vi "2015HEWH_ParseERDInfo.vi"(8 "Error In":errorcluster, 9 "Disable Electronic Mixing Valve (EMV) List":bool, 10 "Disable ERD (Main)":bool, 11 "ERD Data Out":T4[](array[typedef]) {"ERD Number" format="%.0x"}) -> (0 "Error Out":errorcluster, 3 "ERD Data":T1 {"ERD Therm Data"."EEV Possition" format="%0.0f"; "ERD Therm Data"."T6" format="%.1f"; "ERD Therm Data"."T2" format="%.1f"; "ERD Therm Data"."T3a" format="%.1f"; "ERD Therm Data"."T3b" format="%.1f"; "ERD Therm Data"."T4" format="%.1f"; "ERD Therm Data"."T5" format="%.1f"; "ERD Therm Data"."Current" format="%.1f"})   [LabVIEW 2016]
uses:
  type defs/ERD Read Data Out.ctl
  type defs/HEWH ERD Data.ctl
  type defs/HEWH Faults.ctl
  type defs/HEWH Mixing Valve.ctl
  library/GEA2_Toolkit.lvlib
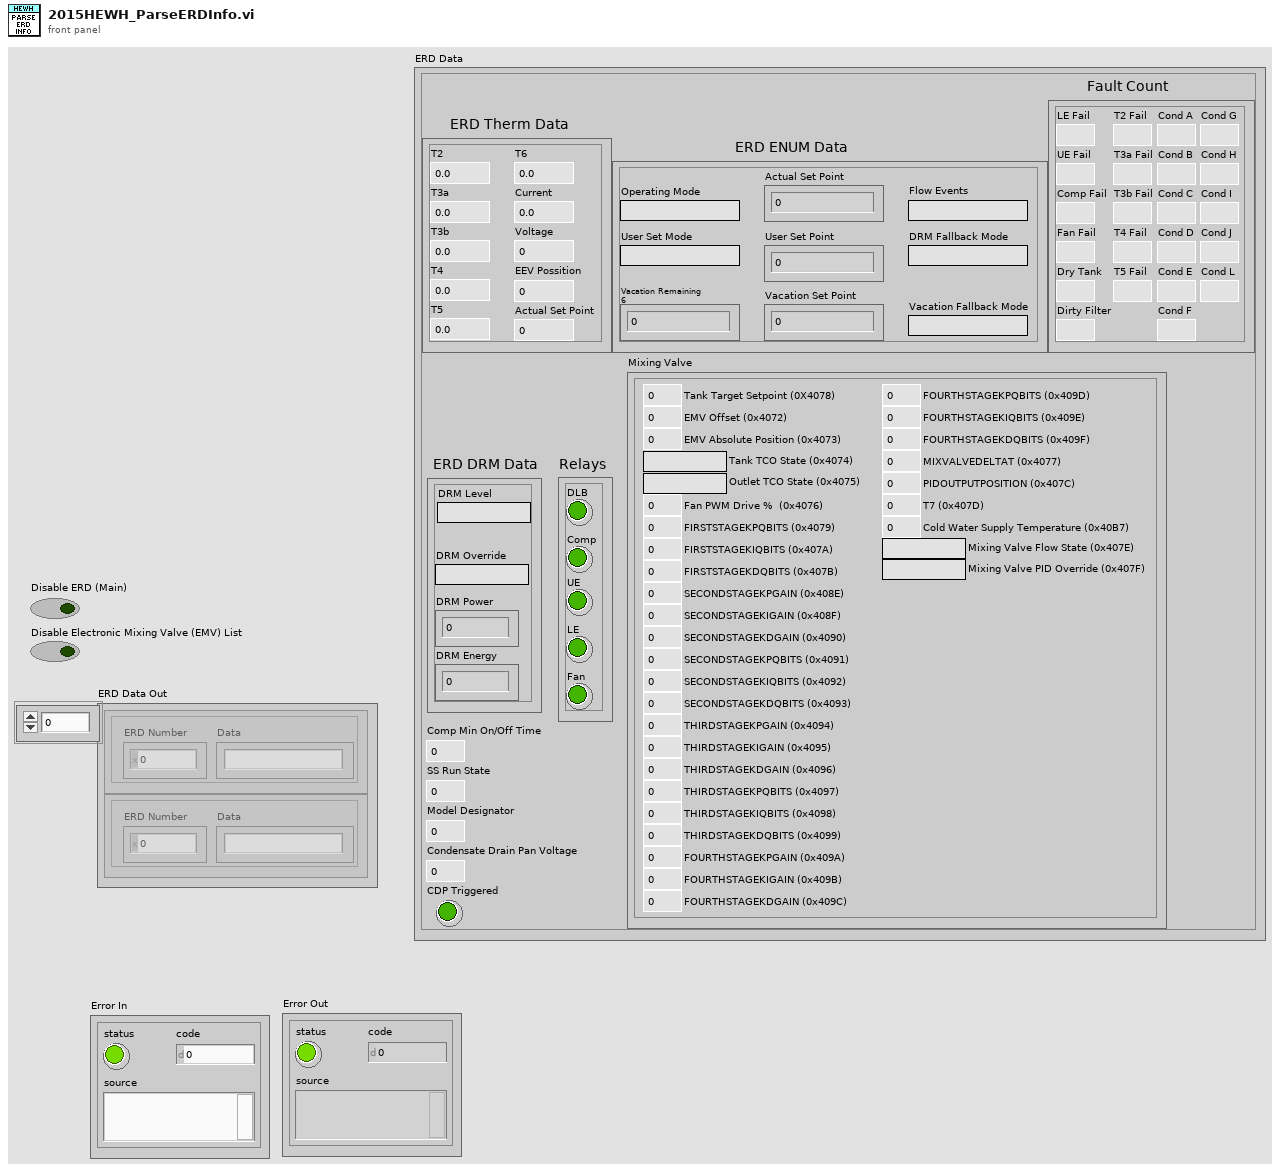
[diagram p1: front panel]
types:
  T1 = typedef "HEWH ERD Data.ctl" = cluster{"ERD Therm Data":cluster{"T2":dbl, "T3a":dbl, "T3b":dbl, "T4":dbl, "T5":dbl, "T6":dbl, "Current":dbl, "Voltage":dbl, "EEV Possition":dbl, "Actual Set Point":dbl}, "ERD ENUM Data":cluster{"Actual Set Point":dbl, "Flow Events":string, "User Set Mode":string, "Operating Mode":string, "DRM Fallback Mode":string, "Vacation Fallback Mode":string, "User Set Point":dbl, "Vacation Set Point":dbl, "Vacation Remaining\n6":dbl}, "ERD DRM Data":cluster{"DRM Level":string, "DRM Override":string, "DRM Power":dbl, "DRM Energy":dbl}, "Fault Count":T2, "Relays":cluster{"DLB":bool, "Comp":bool, "UE":bool, "LE":bool, "Fan":bool}, "Comp Min On/Off Time":u16, "SS Run State":u16, "Condensate Drain Pan Voltage":u16, "CDP Triggered":bool, "Model Designator":u8, "Mixing Valve":T3}
  T2 = typedef "HEWH Faults.ctl" = cluster{"LE Fail":u32, "UE Fail":u32, "Comp Fail":u32, "T2 Fail":u32, "T3a Fail":u32, "T3b Fail":u32, "T4 Fail":u32, "T5 Fail":u32, "Cond A":u32, "Cond B":u32, "Cond C":u32, "Cond D":u32, "Cond E":u32, "Cond F":u32, "Cond G":u32, "Cond H":u32, "Cond I":u32, "Cond J":u32, "Cond L":u32, "Fan Fail":u32, "Dirty Filter":u32, "Dry Tank":u32}
  T3 = typedef "HEWH Mixing Valve.ctl" = cluster{"Tank Target Setpoint (0X4078)":dbl, "EMV Offset (0x4072)":dbl, "EMV Absolute Position (0x4073)":dbl, "Tank TCO State (0x4074)":string, "Outlet TCO State (0x4075)":string, "Fan PWM Drive %  (0x4076)":dbl, "FIRSTSTAGEKPQBITS (0x4079)":dbl, "FIRSTSTAGEKIQBITS (0x407A)":dbl, "FIRSTSTAGEKDQBITS (0x407B)":dbl, "SECONDSTAGEKPGAIN (0x408E)":dbl, "SECONDSTAGEKIGAIN (0x408F)":dbl, "SECONDSTAGEKDGAIN (0x4090)":dbl, "SECONDSTAGEKPQBITS (0x4091)":dbl, "SECONDSTAGEKIQBITS (0x4092)":dbl, "SECONDSTAGEKDQBITS (0x4093)":dbl, "THIRDSTAGEKPGAIN (0x4094)":dbl, "THIRDSTAGEKIGAIN (0x4095)":dbl, "THIRDSTAGEKDGAIN (0x4096)":dbl, "THIRDSTAGEKPQBITS (0x4097)":dbl, "THIRDSTAGEKIQBITS (0x4098)":dbl, "THIRDSTAGEKDQBITS (0x4099)":dbl, "FOURTHSTAGEKPGAIN (0x409A)":dbl, "FOURTHSTAGEKIGAIN (0x409B)":dbl, "FOURTHSTAGEKDGAIN (0x409C)":dbl, "FOURTHSTAGEKPQBITS (0x409D)":dbl, "FOURTHSTAGEKIQBITS (0x409E)":dbl, "FOURTHSTAGEKDQBITS (0x409F)":dbl, "MIXVALVEDELTAT (0x4077)":dbl, "PIDOUTPUTPOSITION (0x407C)":dbl, "T7 (0x407D)":dbl, "Cold Water Supply Temperature (0x40B7)":dbl, "Mixing Valve Flow State (0x407E)":string, "Mixing Valve PID Override (0x407F)":string}
  T4 = typedef "GEA2_Toolkit.lvlib/ERD Read Data Out.ctl" = cluster{"ERD Number":u16, "Data":string}
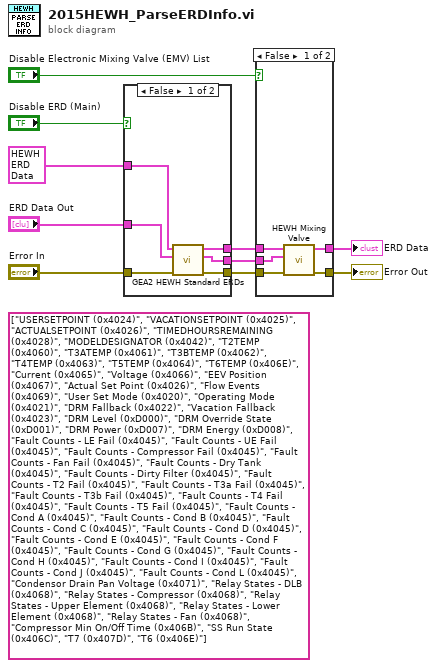
[diagram p0: block diagram]
diagram:
  (unwired) string[] ["USERSETPOINT (0x4024)", "VACATIONSETPOINT (0x4025)", "ACTUALSETPOINT (0x4026)", "TIMEDHOURSREMAINING (0x4028)", "MODELDESIGNATOR (0x4042)", "T2TEMP (0x4060)", "T3ATEMP (0x4061)", "T3BTEMP (0x4062)", "T4TEMP (0x4063)", "T5TEMP (0x4064)", "T6TEMP (0x406E)", "Current (0x4065)", "Voltage (0x4066)", "EEV Position (0x4067)", "Actual Set Point (0x4026)", "Flow Events (0x4069)", "User Set Mode (0x4020)", "Operating Mode (0x4021)", "DRM Fallback (0x4022)", "Vacation Fallback (0x4023)", "DRM Level (0xD000)", "DRM Override State (0xD001)", "DRM Power (0xD007)", "DRM Energy (0xD008)", "Fault Counts - LE Fail (0x4045)", "Fault Counts - UE Fail (0x4045)", "Fault Counts - Compressor Fail (0x4045)", "Fault Counts - Fan Fail (0x4045)", "Fault Counts - Dry Tank (0x4045)", "Fault Counts - Dirty Filter (0x4045)", "Fault Counts - T2 Fail (0x4045)", "Fault Counts - T3a Fail (0x4045)", "Fault Counts - T3b Fail (0x4045)", "Fault Counts - T4 Fail (0x4045)", "Fault Counts - T5 Fail (0x4045)", "Fault Counts - Cond A (0x4045)", "Fault Counts - Cond B (0x4045)", "Fault Counts - Cond C (0x4045)", "Fault Counts - Cond D (0x4045)", "Fault Counts - Cond E (0x4045)", "Fault Counts - Cond F (0x4045)", "Fault Counts - Cond G (0x4045)", "Fault Counts - Cond H (0x4045)", "Fault Counts - Cond I (0x4045)", "Fault Counts - Cond J (0x4045)", "Fault Counts - Cond L (0x4045)", "Condensor Drain Pan Voltage (0x4071)", "Relay States - DLB (0x4068)", "Relay States - Compressor (0x4068)", "Relay States - Upper Element (0x4068)", "Relay States - Lower Element (0x4068)", "Relay States - Fan (0x4068)", "Compressor Min On/Off Time (0x406B)", "SS Run State (0x406C)", "T7 (0x407D)", "T6 (0x406E)"]
  n1 = case shown="False" "Disable ERD (Main)" {
    tunnel: T1 {"ERD Therm Data"={"T2"=0.0, "T3a"=0.0, "T3b"=0.0, "T4"=0.0, "T5"=0.0, "T6"=0.0, "Current"=0.0, "Voltage"=0.0, "EEV Possition"=0.0, "Actual Set Point"=0.0}, "ERD ENUM Data"={"Actual Set Point"=0.0, "Flow Events"="", "User Set Mode"="", "Operating Mode"="", "DRM Fallback Mode"="", "Vacation Fallback Mode"="", "User Set Point"=0.0, "Vacation Set Point"=0.0, "Vacation Remaining\n6"=0.0}, "ERD DRM Data"={"DRM Level"="", "DRM Override"="", "DRM Power"=0.0, "DRM Energy"=0.0}, "Fault Count"={"LE Fail"=0, "UE Fail"=0, "Comp Fail"=0, "T2 Fail"=0, "T3a Fail"=0, "T3b Fail"=0, "T4 Fail"=0, "T5 Fail"=0, "Cond A"=0, "Cond B"=0, "Cond C"=0, "Cond D"=0, "Cond E"=0, "Cond F"=0, "Cond G"=0, "Cond H"=0, "Cond I"=0, "Cond J"=0, "Cond L"=0, "Fan Fail"=0, "Dirty Filter"=0, "Dry Tank"=0}, "Relays"={"DLB"=FALSE, "Comp"=FALSE, "UE"=FALSE, "LE"=FALSE, "Fan"=FALSE}, "Comp Min On/Off Time"=0, "SS Run State"=0, "Condensate Drain Pan Voltage"=0, "CDP Triggered"=FALSE, "Model Designator"=0, "Mixing Valve"={"Tank Target Setpoint (0X4078)"=0.0, "EMV Offset (0x4072)"=0.0, "EMV Absolute Position (0x4073)"=0.0, "Tank TCO State (0x4074)"="", "Outlet TCO State (0x4075)"="", "Fan PWM Drive %  (0x4076)"=0.0, "FIRSTSTAGEKPQBITS (0x4079)"=0.0, "FIRSTSTAGEKIQBITS (0x407A)"=0.0, "FIRSTSTAGEKDQBITS (0x407B)"=0.0, "SECONDSTAGEKPGAIN (0x408E)"=0.0, "SECONDSTAGEKIGAIN (0x408F)"=0.0, "SECONDSTAGEKDGAIN (0x4090)"=0.0, "SECONDSTAGEKPQBITS (0x4091)"=0.0, "SECONDSTAGEKIQBITS (0x4092)"=0.0, "SECONDSTAGEKDQBITS (0x4093)"=0.0, "THIRDSTAGEKPGAIN (0x4094)"=0.0, "THIRDSTAGEKIGAIN (0x4095)"=0.0, "THIRDSTAGEKDGAIN (0x4096)"=0.0, "THIRDSTAGEKPQBITS (0x4097)"=0.0, "THIRDSTAGEKIQBITS (0x4098)"=0.0, "THIRDSTAGEKDQBITS (0x4099)"=0.0, "FOURTHSTAGEKPGAIN (0x409A)"=0.0, "FOURTHSTAGEKIGAIN (0x409B)"=0.0, "FOURTHSTAGEKDGAIN (0x409C)"=0.0, "FOURTHSTAGEKPQBITS (0x409D)"=0.0, "FOURTHSTAGEKIQBITS (0x409E)"=0.0, "FOURTHSTAGEKDQBITS (0x409F)"=0.0, "MIXVALVEDELTAT (0x4077)"=0.0, "PIDOUTPUTPOSITION (0x407C)"=0.0, "T7 (0x407D)"=0.0, "Cold Water Supply Temperature (0x40B7)"=0.0, "Mixing Valve Flow State (0x407E)"="", "Mixing Valve PID Override (0x407F)"=""}} ("ERD Data") -> [w16 w17]
    tunnel: "ERD Data Out" -> [w15 w18]
    tunnel: [w14 w19] -> w8
    tunnel: [w13 w18] -> w7
    tunnel: [w12 w17] -> w6
    tunnel: "Error In" -> [w11 w19]
    frame False {
      n2 = call "GEA2 HEWH Standard ERDs.vi"("Error In"=w11, "ERD Data Input"=w15, "ERD Data  in"=w16) -> ("Error Out"=w14:errorcluster, "ERD Data Output"=w13:T4[], "ERD Data  out"=w12:T1)  [unwired: 6 in]
    }
    frame True {
    }
  }
  n3 = case shown="False" "Disable Electronic Mixing Valve (EMV) List" {
    tunnel: w8 -> [w24 w26]
    tunnel: w7 -> [w23 _]
    tunnel: w6 -> [w22 w25]
    tunnel: [w21 w25] -> w5
    tunnel: [w20 w26] -> w4
    frame False {
      n4 = call "HEWH Mixing Valve.vi"("Error In"=w24, "ERD Data Out"=w23, "ERD Data"=w22) -> ("Error Out"=w20:errorcluster, "ERD Data Out"=w21:T1)  [unwired: 7 in]
    }
    frame True {
    }
  }
  "ERD Data" <- w5
  "Error Out" <- w4
